vi "CalcSpectrum.vi"(6 "WlStop":dbl=340.0, 7 "WlStart":dbl=230.0, 8 "error in (no error)":errorcluster, 10 "Wavelength":dbl[](array[numeric]), 11 "Spectrum":dbl[](array[numeric])) -> (0 "error out":errorcluster, 1 "MaxSpectrum":dbl, 2 "WavelengthSplit":dbl[](array[numeric]), 3 "SpectrumSplit":dbl[](array[numeric]), 4 "Saturated?":bool, 5 "delta":dbl)   [LabVIEW 2012]
panel:
  out "StopIndex":i32
  out "StartIndex":i32
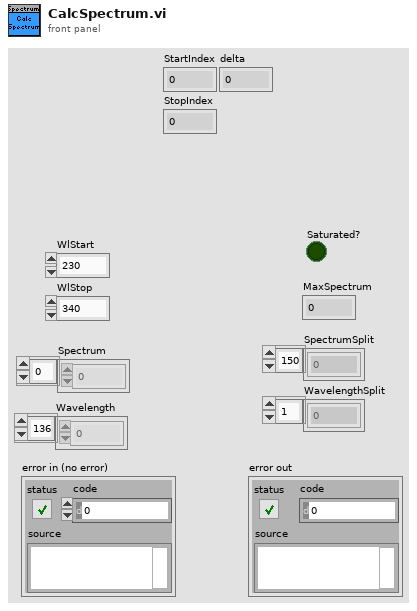
[diagram p1: front panel]
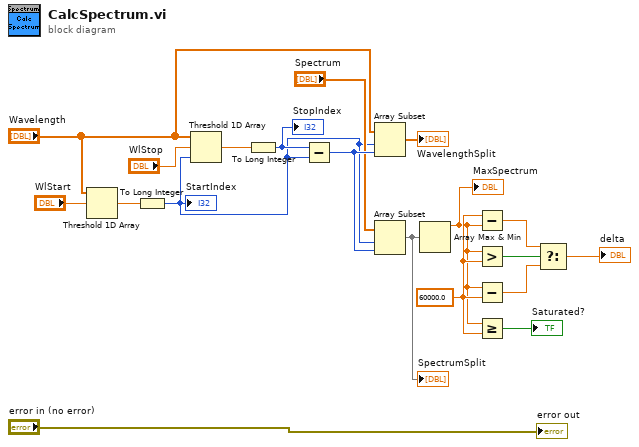
[diagram p0: block diagram]
diagram:
  w4 = 60000.0 ("y")
  n1 = Threshold 1D Array(2:"WlStart", 3:"Wavelength") -> (0:w17:dbl)  [unwired: 1 in]
  n2 = To Long Integer(number=w17) -> (32bit integer=w11:i32)
  "StartIndex" <- w11
  n3 = Threshold 1D Array(1:w11, 2:"WlStop", 3:"Wavelength") -> (0:w16:dbl)
  n4 = To Long Integer(number=w16) -> (32bit integer=w15:i32)
  "StopIndex" <- w15
  n5 = Subtract(x=w15, y=w11) -> (x-y=w14:i32)
  n6 = Array Subset(array="Wavelength", index=w11, length=w14) -> (→"WavelengthSplit":dbl[])
  n7 = Array Subset(array="Spectrum", index=w11, length=w14) -> (w9:dbl[])
  "SpectrumSplit" <- w9
  n8 = Array Max & Min(array=w9) -> (max value=w3:dbl)  [unwired: 3 out]
  "MaxSpectrum" <- w3
  n9 = Subtract(x=w4, y=w3) -> (x-y=w2:dbl)
  n10 = Greater?(x=w3, y=w4) -> (0:w6:bool)
  n11 = Subtract(x=w3, y=w4) -> (x-y=w5:dbl)
  n12 = Greater Or Equal?(x=w3, y=w4) -> (x >= y?=→"Saturated?":bool)
  n13 = Select(t=w2, s=w6, f=w5) -> (s? t:f=→"delta":dbl)
  "error out" <- "error in (no error)"
